vi "Has Value Field.vi"(11 "Option in":refnum<class "Option.lvclass">) -> (2 "Has Value Field":bool, 3 "Option out":refnum<class "Option.lvclass">)   [LabVIEW 2011, in "Option Parser.lvlib" / "Option.lvclass"]
uses:
  Option.lvclass
  Option.lvclass/Option.ctl
  Argument Type.ctl
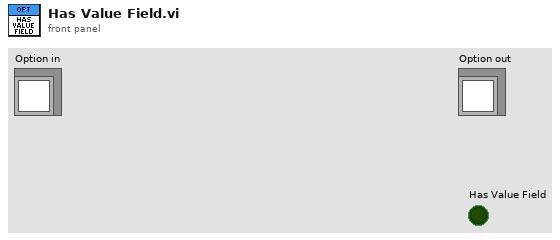
[diagram p1: front panel]
types:
  T1 = typedef "Option Parser.lvlib/Option.lvclass/Argument Type.ctl" = enum16{"flag", "value"}
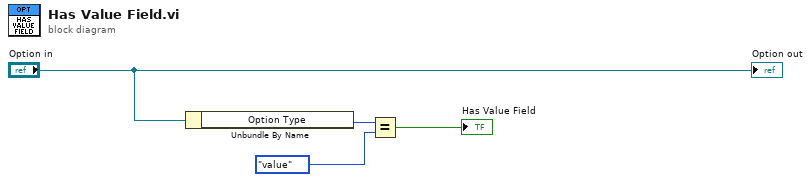
[diagram p0: block diagram]
diagram:
  n1 = Unbundle By Name("Option in") -> ("Option Type"=w3:T1)
  n2 = Equal?(x=w3, y=Argument_Type."value") -> (x = y?=→"Has Value Field":bool)
  "Option out" <- "Option in"
